vi "SeqMgr.Update Progress.vi"(8 "error in":errorcluster, 9 "Result Info":T1={"State"=enum."PASS", "Code"=0, "Description"=""}, 11 "SeqMgr in":refnum<class "SeqMgr.lvclass">) -> (0 "error out":errorcluster, 1 "Result Info Out":T1={"State"=enum."PASS", "Code"=0, "Description"=""}, 2 "Test State":enum32{"Idle", "Running", "Completed"}(ring), 3 "SeqMgr out":refnum<class "SeqMgr.lvclass">, 4 "New Step":string[](array[string]), 5 "Canceled":bool, 6 "StepCnt":i32)   [LabVIEW 2024, in "EQMF.lvlib" / "SeqMgr.lvlib" / "SeqMgr.lvclass"]
uses:
  SeqMgr.lvclass
  SeqMgr.Result Info.ctl
  SeqMgr.Result State Enum.ctl
  SeqMgr.lvclass/SeqMgr.ctl
  SeqMgr.Progress Type.ctl
  <vilib>/Utility/error.llb/Trim Whitespace One-Sided.vi
  SeqMgr.lvlib
  Strings/String Utils.lvlib
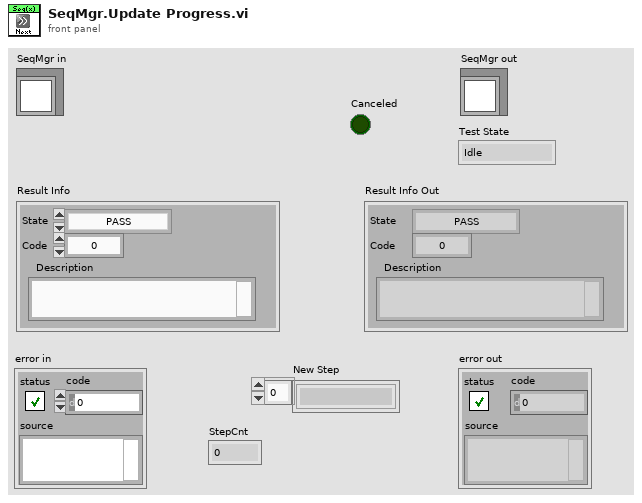
[diagram p1: front panel]
types:
  T1 = typedef "EQMF.lvlib/SeqMgr.lvlib/SeqMgr.Result Info.ctl" = cluster{"State":T2, "Code":i32, "Description":string}
  T2 = typedef "EQMF.lvlib/SeqMgr.lvlib/SeqMgr.Result State Enum.ctl" = enum16{"None", "Passing", "Failing", "PASS", "FAIL", "ABORT", "ERROR"}
  T3 = typedef "EQMF.lvlib/SeqMgr.lvlib/SeqMgr.Progress Type.ctl" = enum16{"Steps", "Time"}
  T4 = typedef "EQMF.lvlib/SeqMgr.lvlib/SeqMgr.Progress Info.ctl" = cluster{"Running":bool, "StartTime":timestamp, "EndTime":timestamp, "Progress":dbl, "Duration(s)":dbl, "ProgType":T3, "StepCnt":i32, "StepTotal":i32, "RemainingTime(s)":dbl, "Test State":enum32{"Idle", "Running", "Completed"}}
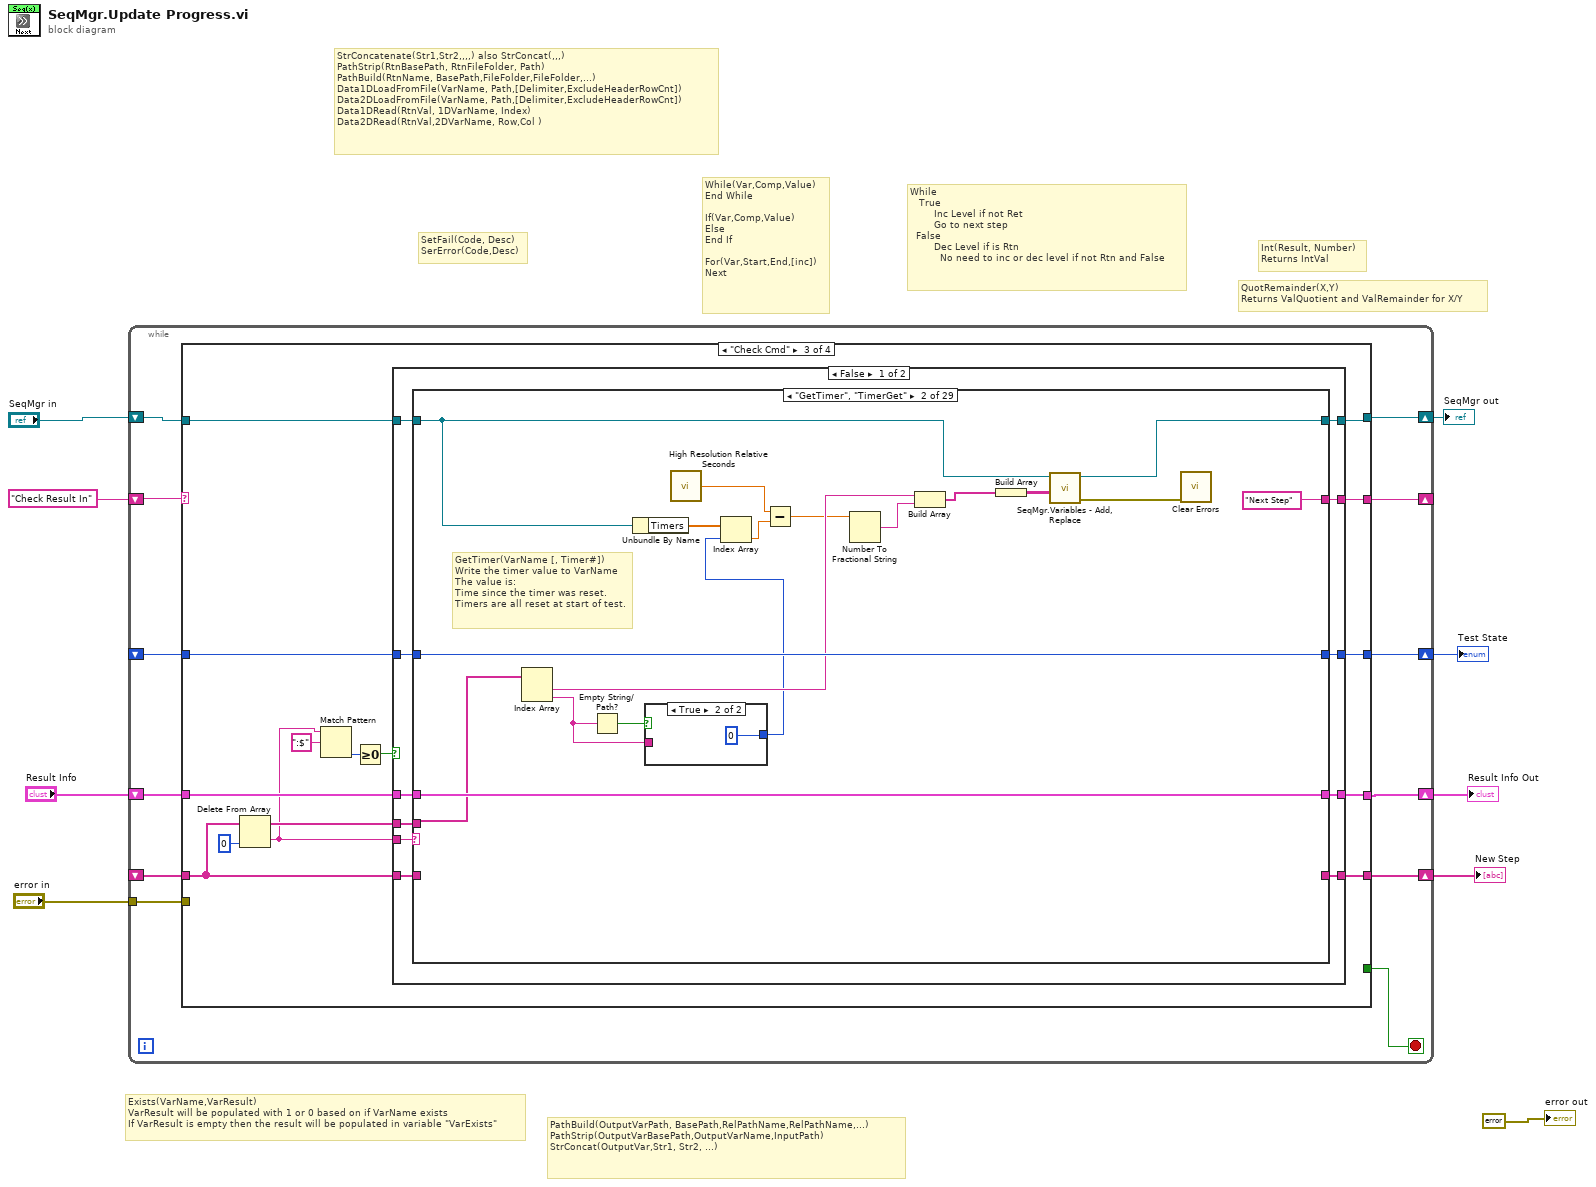
[diagram p0: block diagram]
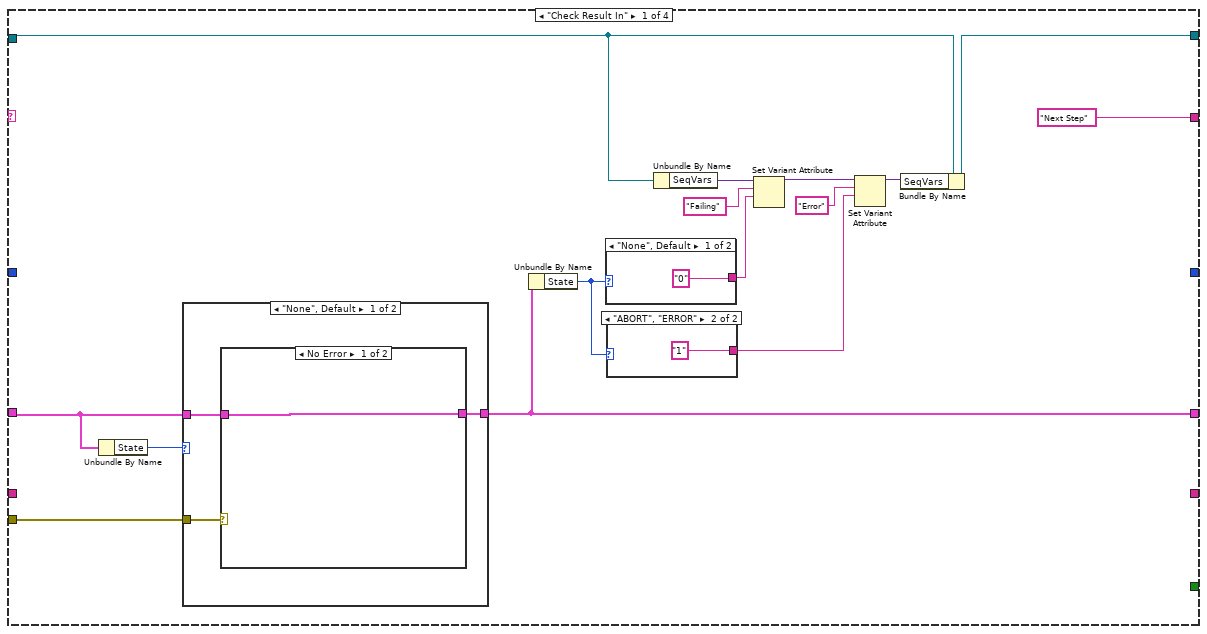
[diagram p2: hidden frame]
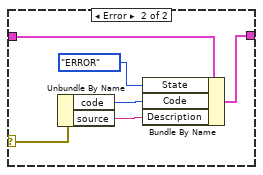
[diagram p3: hidden frame]
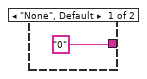
[diagram p5: hidden frame]
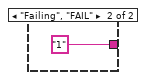
[diagram p6: hidden frame]
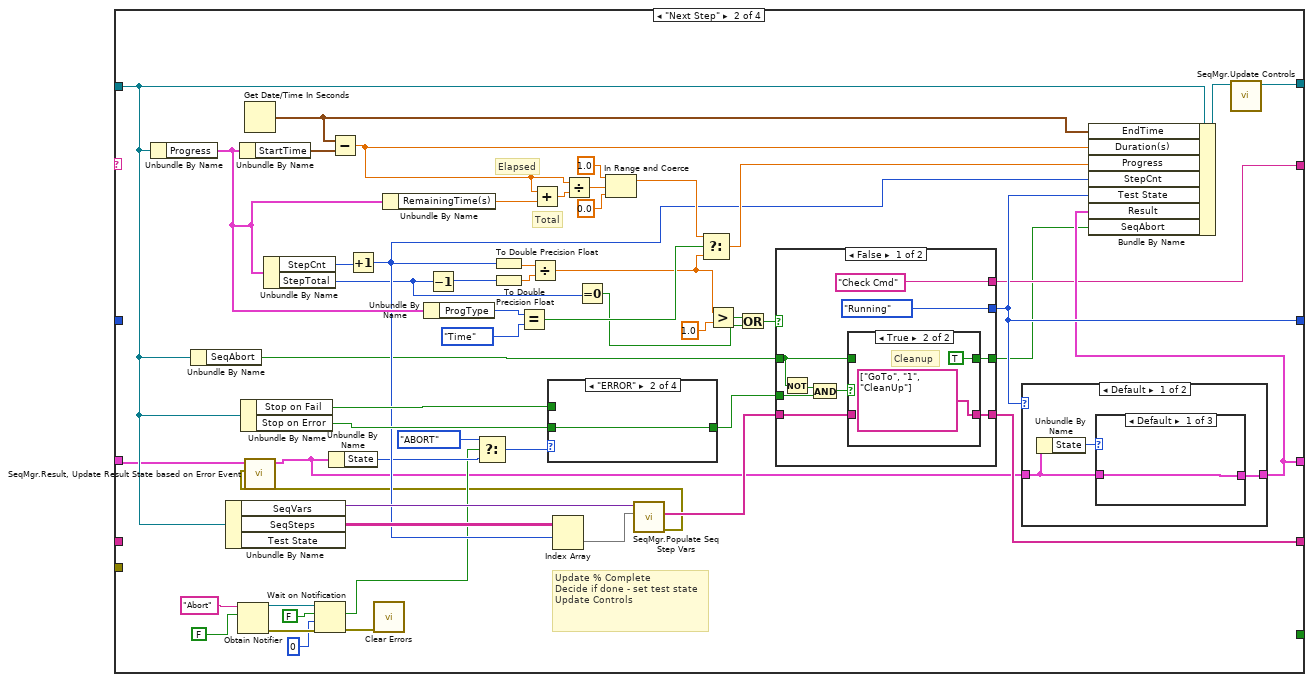
[diagram p7: hidden frame]
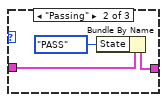
[diagram p8: hidden frame]
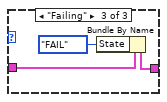
[diagram p9: hidden frame]
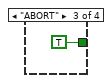
[diagram p12: hidden frame]
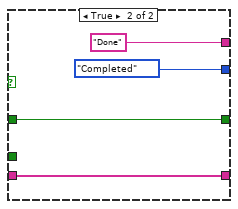
[diagram p15: hidden frame]
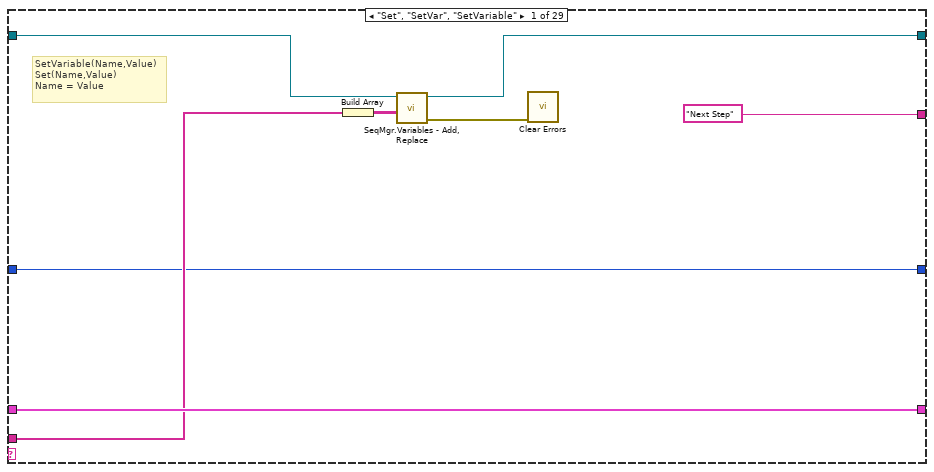
[diagram p16: hidden frame]
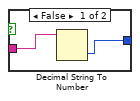
[diagram p17: hidden frame]
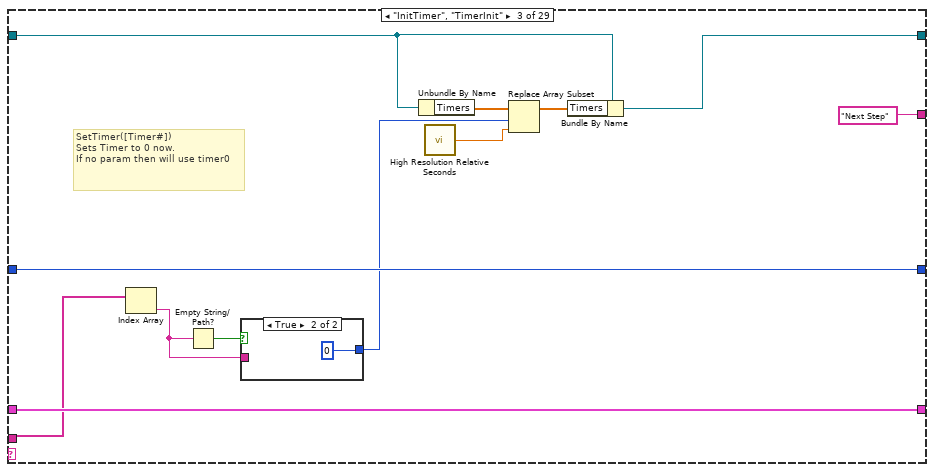
[diagram p18: hidden frame]
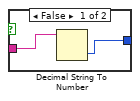
[diagram p19: hidden frame]
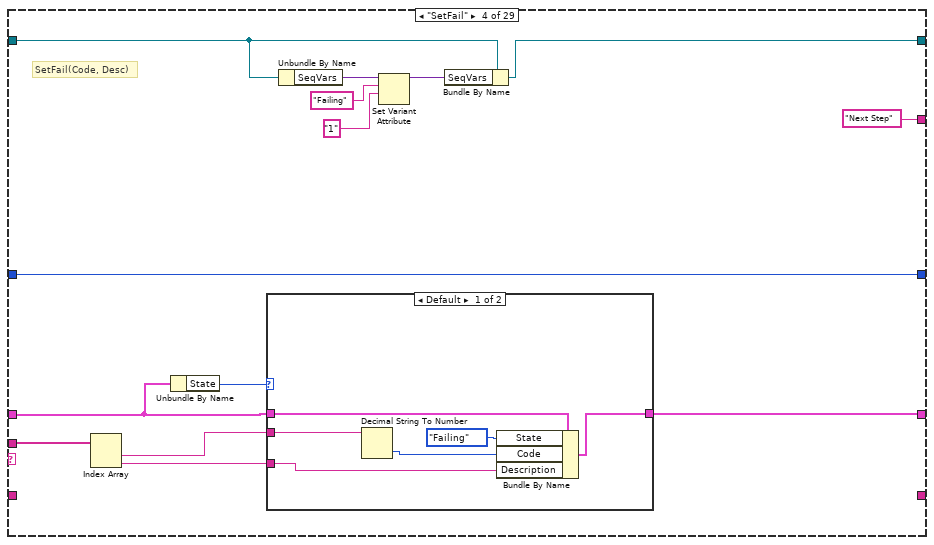
[diagram p20: hidden frame]
diagram:
  # "Exists(VarName,VarResult)\nVarResult will be populated with 1 or 0 based on if VarName exists\nIf VarResult is empty then the result will be populated in variable \"VarExists\""
  # "QuotRemainder(X,Y)\nReturns ValQuotient and ValRemainder for X/Y"
  # "Int(Result, Number)\nReturns IntVal"
  # "StrConcatenate(Str1,Str2,,,,) also StrConcat(,,,)\nPathStrip(RtnBasePath, RtnFileFolder, Path)\nPathBuild(RtnName, BasePath,FileFolder,FileFolder,...)\nData1DLoadFromFile(VarName, Path,[Delimiter,ExcludeHeaderRowCnt])\nData2DLoadFromFile(VarName, Path,[Delimiter,ExcludeHeaderRowCnt])\nData1DRead(RtnVal, 1DVarName, Index)\nData2DRead(RtnVal,2DVarName, Row,Col )"
  # "PathBuild(OutputVarPath, BasePath,RelPathName,RelPathName,...)\nPathStrip(OutputVarBasePath,OutputVarName,InputPath)\nStrConcat(OutputVar,Str1, Str2, ...)"
  # "SetFail(Code, Desc)\nSerError(Code,Desc)"
  # "While\n   True\n        Inc Level if not Ret\n        Go to next step\n  False\n        Dec Level if is Rtn\n          No need to inc or dec level if not Rtn and False"
  # "While(Var,Comp,Value)\nEnd While\n\nIf(Var,Comp,Value)\nElse\nEnd If\n\nFor(Var,Start,End,[inc])\nNext"
  n1 = while {
    shift-right: [w20] -> w8
    shift-left: "SeqMgr in" -> [w21]
    shift-right: [w17] -> w5
    shift-left: "Result Info" -> [w16]
    shift-right: [w13] -> _
    shift-left: "Check Result In" -> [w15]
    tunnel: "error in" -> [w14]
    shift-right: [w19] -> w7
    shift-left: _ -> [w11]
    shift-right: [w18] -> w6
    shift-left: _ -> [w12]
    stop <- w10 stop-if-true
    n2 = case shown="\"Check Cmd\"" w15 {
      tunnel: w21 -> [w32 w67 w152 w914]
      tunnel: [w31 w106 w151 w915] -> w20
      tunnel: [_ w70 w143 w929] -> w19
      tunnel: [_ w105 w146 w930] -> w18
      tunnel: [w27 w104 w145 w916] -> w17
      tunnel: w16 -> [w23 w53 w148 w916]
      tunnel: w14 -> [w36 _ _ _]
      tunnel: ["Next Step" w73 w142 "Done"] -> w13
      tunnel: w12 -> [_ _ w147 w930]
      tunnel: w11 -> [_ _ w144 w929]
      tunnel: [_ _ _ TRUE] -> w10
      frame "Check Result In" {
        n3 = Unbundle By Name(w23) -> ("State"=w22:T2)
        n4 = case shown="\"None\", Default" w22 {
          tunnel: w36 -> [w39 _]
          tunnel: w23 -> [w38 w47]
          tunnel: [w37 w47] -> w27
          frame "None", Default {
            n5 = case shown="No Error" w39 {
              selector: w39 -> [_ w43]
              tunnel: w38 -> [w40 w46]
              tunnel: [w40 w45] -> w37
              frame No Error {
              }
              frame Error {
                n6 = Unbundle By Name(w43) -> ("code"=w42:i32, "source"=w41:string)
                n7 = Bundle By Name(cluster=w46, "State"=SeqMgr.Result_State_Enum."ERROR", "Code"=w42, "Description"=w41) -> (w45:T1)
              }
            }
          }
          frame "ABORT", "ERROR" {
          }
        }
        n8 = Unbundle By Name(w27) -> ("State"=w26:T2)
        n9 = case shown="\"None\", Default" w26 {
          tunnel: ["0" "1"] -> w30
          frame "None", Default {
          }
          frame "Failing", "FAIL" {
          }
        }
        n10 = case shown="\"ABORT\", \"ERROR\"" w26 {
          tunnel: ["0" "1"] -> w25
          frame "None", Default {
          }
          frame "ABORT", "ERROR" {
          }
        }
        n11 = Unbundle By Name(w32) -> ("SeqVars"=w33:variant)
        n12 = Set Variant Attribute(Variant=w33, name="Failing", value=w30) -> (Variant out=w29:variant)  [unwired: 1 in, 2 out]
        n13 = Set Variant Attribute(Variant=w29, name="Error", value=w25) -> (Variant out=w28:variant)  [unwired: 1 in, 2 out]
        n14 = Bundle By Name(cluster=w32, "SeqVars"=w28) -> (w31:refnum<class "SeqMgr.lvclass">)
      }
      frame "Next Step" {
        # "Elapsed"
        # "Total"
        # "Update % Complete\nDecide if done - set test state\nUpdate Controls"
        n15 = Unbundle By Name(w67) -> ("Progress"=w88:T4)
        n16 = Unbundle By Name(w67) -> ("SeqAbort"=w66:bool)
        n17 = Unbundle By Name(w67) -> ("SeqVars"=w79:variant, "SeqSteps"=w87:string[][])  [unwired: 1 out]
        n18 = Obtain Notifier(name (unnamed)="Abort", notification data type=FALSE ("create if not found? (T)")) -> (notifier out=w62:refnum<notifier>, error out=w61:errorcluster)  [unwired: 2 in, 1 out]
        n19 = Unbundle By Name(w88) -> ("StartTime"=w103:timestamp)
        n20 = Unbundle By Name(w67) -> ("Stop on Fail"=w81:bool, "Stop on Error"=w80:bool)
        n21 = Get Date/Time In Seconds() -> (seconds since 1Jan1904=w72:timestamp)
        n22 = Unbundle By Name(w88) -> ("StepCnt"=w89:i32, "StepTotal"=w75:i32)
        n23 = Wait on Notification(notifier=w62, ignore previous (F)=FALSE, timeout in ms (-1)=0, error in (no error)=w61) -> (notification=w55:bool, error out=w60:errorcluster)  [unwired: 2 out]
        n24 = Subtract(x=w72, y=w103) -> (x-y=w102:dbl)
        n25 = Increment(x=w89) -> (x+1=w77:i32)
        n26 = call <vilib>:"Clear Errors.vi"("error in (no error)"=w60) -> ()  [unwired: 5 in, 2 out]
        n27 = Unbundle By Name(w88) -> ("RemainingTime(s)"=w99:dbl)
        n28 = Unbundle By Name(w88) -> ("ProgType"=w93:T3)
        n29 = Decrement(x=w75) -> (x-1=w76:i32)
        n30 = To Double Precision Float(number=w77) -> (double precision float=w100:dbl)
        n31 = To Double Precision Float(number=w76) -> (double precision float=w101:dbl)
        n32 = Equal?(x=w93, y=SeqMgr.Progress_Type."Time" ("ProgType")) -> (x = y?=w91:bool)
        n33 = Divide(x=w100, y=w101) -> (x/y=w86:dbl)
        n34 = Add(x=w102, y=w99) -> (x+y=w98:dbl)
        n35 = Index Array(array=w87, index (row)=w77) -> (element=w78:string[])  [unwired: 1 in]
        n36 = Divide(x=w102, y=w98) -> (x/y=w97:dbl)
        n37 = Equal To 0?(x=w75) -> (x = 0?=w74:bool)
        n38 = In Range and Coerce(upper limit=1.0, x=w97, lower limit=0.0 ("upper limit")) -> (coerced(x)=w94:dbl)  [unwired: 1 out]
        n39 = call "SeqMgr.Populate Seq Step Vars.vi"("Seq Step In"=w78, "Variable Values"=w79) -> ("error out"=w52:errorcluster, "Seq Step Out"=w71:string[])  [unwired: 8 in]
        n40 = call "SeqMgr.Result, Update Result State based on Error Event.vi"("error in"=w52, "Result Info"=w53) -> ("Result Info Out"=w54:T1)  [unwired: 9 in]
        n41 = Unbundle By Name(w54) -> ("State"=w65:T2)
        n42 = Select(t=SeqMgr.Result_State_Enum."ABORT", s=w55, f=w65) -> (s? t:f=w64:T2)
        n43 = case shown="\"ERROR\"" w64 {
          tunnel: w81 -> [w118 _ _ _]
          tunnel: w80 -> [_ w119 _ _]
          tunnel: [w118 w119 TRUE _] -> w69
          frame "Failing", "FAIL" {
          }
          frame "ERROR" {
          }
          frame "ABORT" {
          }
          frame "Passing", Default {
          }
        }
        n44 = Select(t=w94, s=w91, f=w86) -> (s? t:f=w90:dbl)
        n45 = Greater?(x=w86, y=1.0 ("upper limit")) -> (0:w83:bool)
        n46 = Or(x=w83, y=w74) -> (x .or. y?=w84:bool)
        n47 = case shown="False" w84 {
          tunnel: [enum32{"Idle", "Running", "Completed"}."Running" ("Progress.Test State") enum32{"Idle", "Running", "Completed"}."Completed" ("Progress.Test State")] -> w105
          tunnel: ["Check Cmd" "Done"] -> w73
          tunnel: w71 -> [w126 w135]
          tunnel: [w127 w135] -> w70
          tunnel: w69 -> [w125 _]
          tunnel: [w123 w134] -> w68
          tunnel: w66 -> [w121 w134]
          frame False {
            n48 = Not(x=w121) -> (.not. x?=w122:bool)
            n49 = And(x=w122, y=w125) -> (x .and. y?=w124:bool)
            n50 = case shown="True" w124 {
              tunnel: [w131 string[] ["GoTo", "1", "CleanUp"]] -> w127
              tunnel: w126 -> [w131 _]
              tunnel: [w130 TRUE] -> w123
              tunnel: w121 -> [w130 _]
              frame False {
              }
              frame True {
                # "Cleanup"
              }
            }
          }
          frame True {
          }
        }
        n51 = case shown="Default" w105 {
          tunnel: w54 -> [w107 w117]
          tunnel: [w108 w117] -> w104
          frame Default {
            n52 = Unbundle By Name(w107) -> ("State"=w109:T2)
            n53 = case shown="Default" w109 {
              tunnel: [w110 w113 w116] -> w108
              tunnel: w107 -> [w110 w112 w115]
              frame Default {
              }
              frame "Passing" {
                n54 = Bundle By Name(cluster=w112, "State"=SeqMgr.Result_State_Enum."PASS") -> (w113:T1)
              }
              frame "Failing" {
                n55 = Bundle By Name(cluster=w115, "State"=SeqMgr.Result_State_Enum."FAIL") -> (w116:T1)
              }
            }
          }
          frame "Running" {
          }
        }
        n56 = Bundle By Name(cluster=w67, "EndTime"=w72, "Duration(s)"=w102, "Progress"=w90, "StepCnt"=w77, "Test State"=w105, "Result"=w104, "SeqAbort"=w68) -> (w82:refnum<class "SeqMgr.lvclass">)
        n57 = call "SeqMgr.Update Controls.vi"("SeqMgr in"=w82) -> ("SeqMgr out"=w106:refnum<class "SeqMgr.lvclass">)  [unwired: 9 in, 1 out]
      }
      frame "Check Cmd" {
        n58 = Delete From Array(array=w144, index=0) -> (deleted portion=w140:string, array with subset deleted=w149:string[])  [unwired: 1 in]
        n59 = Match Pattern(string=w140, regular expression=":$") -> (offset past match=w139:i32)  [unwired: 1 in, 3 out]
        n60 = Greater Or Equal To 0?(x=w139) -> (x >= 0?=w138:bool)
        n61 = case shown="False" w138 {
          tunnel: w152 -> [w163 w913]
          tunnel: [w162 w913] -> w151
          tunnel: w149 -> [w161 _]
          tunnel: w148 -> [w160 w911]
          tunnel: w147 -> [w159 w912]
          tunnel: [w158 w912] -> w146
          tunnel: [w157 w911] -> w145
          tunnel: w144 -> [w156 w910]
          tunnel: [w155 w910] -> w143
          tunnel: [w154 "Next Step"] -> w142
          tunnel: w140 -> [w153 _]
          frame False {
            n62 = case shown="\"GetTimer\", \"TimerGet\"" w153 {
              tunnel: w163 -> [w168 w181 w196 w215 w236 w255 w270 w284 w305 w312 w319 w356 w385 w422 w479 w495 w529 w599 w614 w707 w722 w755 w768 w783 w811 w833 w861 w897 w908]
              tunnel: [w167 w186 w195 w214 w235 w254 w269 w283 w304 w313 w318 w355 w384 w429 w478 w504 w539 w598 w624 w706 w721 w754 w767 w782 w810 w832 w860 w898 w908] -> w162
              tunnel: w161 -> [w166 w180 w201 w210 w231 w251 w266 w280 w301 w311 w327 w364 w383 w424 _ w494 w534 _ w611 _ w725 w751 w763 w781 w809 w844 w870 w894 _]
              tunnel: w160 -> [w170 w188 w203 w213 w234 w256 w271 w285 w306 w314 w321 w358 w387 w431 w474 w500 w541 w591 w626 w700 w728 w758 w771 w777 w805 w848 w874 w895 w906]
              tunnel: w159 -> [w164 w184 w202 w220 w241 w252 w267 w281 w302 w309 w322 w359 w388 w432 w472 w498 w542 w592 w627 w699 w726 w756 w769 w784 w812 w849 w875 w893 w907]
              tunnel: [w164 w184 w202 w220 w241 w252 w267 w281 w302 w309 w324 w361 w390 w433 w472 w498 w543 w592 w628 w699 w726 w756 w769 w784 w812 w849 w875 w893 w907] -> w158
              tunnel: [w170 w188 w203 w211 w232 w256 w271 w285 w306 w314 w320 w357 w386 w430 w473 w499 w540 w594 w625 w701 w728 w758 w771 w776 w804 w847 w873 w895 w906] -> w157
              tunnel: w156 -> [_ _ _ _ _ _ _ _ _ _ _ _ _ _ _ _ _ _ _ _ _ _ _ _ _ _ _ _ w905]
              tunnel: [_ _ _ _ _ _ _ _ _ _ _ _ _ _ _ _ _ _ _ _ _ _ _ _ _ _ _ _ w905] -> w155
              tunnel: ["Next Step" "Next Step" "Next Step" "Next Step" "Next Step" "Next Step" "Next Step" "Next Step" "Next Step" "Next Step" w328 w365 w393 "Next Step" "Next Step" "Next Step" "Next Step" "Next Step" "Next Step" "Next Step" "Next Step" "Next Step" "Next Step" "Next Step" "Next Step" "Next Step" "Next Step" "Next Step" "Done"] -> w154
              frame "Set", "SetVar", "SetVariable" {
                # "SetVariable(Name,Value)\nSet(Name,Value)\nName = Value"
                n63 = Build Array(w166) -> (w169:string[][])
                n64 = call "SeqMgr.Variables - Add, Replace.vi"("Name, Value"=w169, "SeqMgr in"=w168) -> ("error out"=w165:errorcluster, "SeqMgr out"=w167:refnum<class "SeqMgr.lvclass">)  [unwired: 8 in]
                n65 = call <vilib>:"Clear Errors.vi"("error in (no error)"=w165) -> ()  [unwired: 5 in, 2 out]
              }
              frame "GetTimer", "TimerGet" {
                # "GetTimer(VarName [, Timer#])\nWrite the timer value to VarName\nThe value is:\nTime since the timer was reset.\nTimers are all reset at start of test."
                n66 = Index Array(array=w180) -> (element #1=w176:string, element #2=w178:string)  [unwired: 2 in]
                n67 = Empty String/Path?(string/path=w178) -> (empty?=w179:bool)
                n68 = Unbundle By Name(w181) -> ("Timers"=w177:dbl[])
                n69 = case shown="True" w179 {
                  tunnel: w178 -> [w191 _]
                  tunnel: [w190 0] -> w172
                  frame False {
                    n70 = Decimal String To Number(string=w191) -> (number=w190:i32)  [unwired: 2 in, 1 out]
                  }
                  frame True {
                  }
                }
                n71 = call <vilib>:"High Resolution Relative Seconds.vi"() -> ("relative seconds"=w175:dbl)
                n72 = Index Array(array=w177, index=w172) -> (element=w174:dbl)
                n73 = Subtract(x=w175, y=w174) -> (x-y=w173:dbl)
                n74 = Number To Fractional String(number=w173) -> (F-format string=w182:string)  [unwired: 3 in]
                n75 = Build Array(w176, w182) -> (w183:string[])
                n76 = Build Array(w183) -> (w187:string[][])
                n77 = call "SeqMgr.Variables - Add, Replace.vi"("Name, Value"=w187, "SeqMgr in"=w181) -> ("error out"=w185:errorcluster, "SeqMgr out"=w186:refnum<class "SeqMgr.lvclass">)  [unwired: 8 in]
                n78 = call <vilib>:"Clear Errors.vi"("error in (no error)"=w185) -> ()  [unwired: 5 in, 2 out]
              }
              frame "InitTimer", "TimerInit" {
                # "SetTimer([Timer#])\nSets Timer to 0 now.\nIf no param then will use timer0"
                n79 = Index Array(array=w201) -> (element=w197:string)  [unwired: 1 in]
                n80 = Empty String/Path?(string/path=w197) -> (empty?=w200:bool)
                n81 = case shown="True" w200 {
                  tunnel: w197 -> [w206 _]
                  tunnel: [w205 0] -> w198
                  frame False {
                    n82 = Decimal String To Number(string=w206) -> (number=w205:i32)  [unwired: 2 in, 1 out]
                  }
                  frame True {
                  }
                }
                n83 = Unbundle By Name(w196) -> ("Timers"=w199:dbl[])
                n84 = call <vilib>:"High Resolution Relative Seconds.vi"() -> ("relative seconds"=w193:dbl)
                n85 = Replace Array Subset(array=w199, new element=w193, index=w198) -> (w194:dbl[])
                n86 = Bundle By Name(cluster=w196, "Timers"=w194) -> (w195:refnum<class "SeqMgr.lvclass">)
              }
              frame "SetFail" {
                # "SetFail(Code, Desc)"
                n87 = Index Array(array=w210) -> (element #1=w209:string, element #2=w208:string)  [unwired: 2 in]
                n88 = Unbundle By Name(w213) -> ("State"=w212:T2)
                n89 = case shown="Default" w212 {
                  tunnel: w213 -> [w227 w228]
                  tunnel: [w226 w228] -> w211
                  tunnel: w209 -> [w224 _]
                  tunnel: w208 -> [w223 _]
                  frame Default {
                    n90 = Decimal String To Number(string=w224) -> (number=w222:i32)  [unwired: 2 in, 1 out]
                    n91 = Bundle By Name(cluster=w227, "State"=SeqMgr.Result_State_Enum."Failing", "Code"=w222, "Description"=w223) -> (w226:T1)
                  }
                  frame "Failing", "FAIL", "ERROR" {
                    # "No Change"
                  }
                }
                n92 = Unbundle By Name(w215) -> ("SeqVars"=w217:variant)
                n93 = Set Variant Attribute(Variant=w217, name="Failing", value="1") -> (Variant out=w218:variant)  [unwired: 1 in, 2 out]
                n94 = Bundle By Name(cluster=w215, "SeqVars"=w218) -> (w214:refnum<class "SeqMgr.lvclass">)
              }
              frame "SetError" {
                # "SetError(Code, Desc)"
                n95 = Index Array(array=w231) -> (element #1=w230:string, element #2=w229:string)  [unwired: 2 in]
                n96 = Unbundle By Name(w234) -> ("State"=w233:T2)
                n97 = case shown="Default" w233 {
                  tunnel: w234 -> [w248 w249]
                  tunnel: [w247 w249] -> w232
                  tunnel: w230 -> [w245 _]
                  tunnel: w229 -> [w244 _]
                  frame Default {
                    n98 = Decimal String To Number(string=w245) -> (number=w243:i32)  [unwired: 2 in, 1 out]
                    n99 = Bundle By Name(cluster=w248, "State"=SeqMgr.Result_State_Enum."ERROR", "Code"=w243, "Description"=w244) -> (w247:T1)
                  }
                  frame "ERROR" {
                    # "No Change"
                  }
                }
                n100 = Unbundle By Name(w236) -> ("SeqVars"=w238:variant)
                n101 = Set Variant Attribute(Variant=w238, name="Error", value="1") -> (Variant out=w239:variant)  [unwired: 1 in, 2 out]
                n102 = Bundle By Name(cluster=w236, "SeqVars"=w239) -> (w235:refnum<class "SeqMgr.lvclass">)
              }
              frame "Math" {
                # "Math(Result,Value1,Oper,Value2)\nName = Value Oper Value"
                n103 = call "SeqMgr.Math Statement Execute.vi"("Arguements"=w251) -> ("Vars Out"=w250:string[][])  [unwired: 10 in]
                n104 = call "SeqMgr.Variables - Add, Replace.vi"("Name, Value"=w250, "SeqMgr in"=w255) -> ("error out"=w253:errorcluster, "SeqMgr out"=w254:refnum<class "SeqMgr.lvclass">)  [unwired: 8 in]
                n105 = call <vilib>:"Clear Errors.vi"("error in (no error)"=w253) -> ()  [unwired: 5 in, 2 out]
              }
              frame "Int" {
                n106 = Index Array(array=w266) -> (element #1=w263:string, element #2=w265:string)  [unwired: 2 in]
                n107 = Fract/Exp String To Number(string=w265) -> (number=w259:dbl)  [unwired: 3 in, 1 out]
                n108 = Round To Nearest(number=w259) -> (nearest integer value=w258:dbl)
                n109 = To Long Integer(number=w258) -> (32bit integer=w264:i32)
                n110 = Number To Decimal String(number=w264) -> (decimal integer string=w262:string)  [unwired: 1 in]
                n111 = Build Array(w263, w262) -> (w261:string[])
                n112 = Build Array(w261) -> (w260:string[][])
                n113 = call "SeqMgr.Variables - Add, Replace.vi"("Name, Value"=w260, "SeqMgr in"=w270) -> ("error out"=w268:errorcluster, "SeqMgr out"=w269:refnum<class "SeqMgr.lvclass">)  [unwired: 8 in]
                n114 = call <vilib>:"Clear Errors.vi"("error in (no error)"=w268) -> ()  [unwired: 5 in, 2 out]
              }
              frame "AbsVal" {
                n115 = Index Array(array=w280) -> (element #1=w278:string, element #2=w279:string)  [unwired: 2 in]
                n116 = Fract/Exp String To Number(string=w279) -> (number=w275:dbl)  [unwired: 3 in, 1 out]
                n117 = Absolute Value(x=w275) -> (abs(x)=w274:dbl)
                n118 = call "String.Float to String, No Trailing Zeros.vi"("Numeric"=w274) -> ("String"=w273:string)  [unwired: 10 in]
                n119 = Build Array(w278, w273) -> (w277:string[])
                n120 = Build Array(w277) -> (w276:string[][])
                n121 = call "SeqMgr.Variables - Add, Replace.vi"("Name, Value"=w276, "SeqMgr in"=w284) -> ("error out"=w282:errorcluster, "SeqMgr out"=w283:refnum<class "SeqMgr.lvclass">)  [unwired: 8 in]
                n122 = call <vilib>:"Clear Errors.vi"("error in (no error)"=w282) -> ()  [unwired: 5 in, 2 out]
              }
              frame "QuotRemainder" {
                n123 = Index Array(array=w301) -> (element #1=w300:string, element #2=w297:string)  [unwired: 2 in]
                n124 = Fract/Exp String To Number(string=w297) -> (number=w295:dbl)  [unwired: 3 in, 1 out]
                n125 = Fract/Exp String To Number(string=w300) -> (number=w296:dbl)  [unwired: 3 in, 1 out]
                n126 = Quotient & Remainder(x=w296, y=w295) -> (x-y*floor(x/y)=w294:dbl, floor(x/y)=w292:dbl)
                n127 = To Long Integer(number=w292) -> (32bit integer=w293:i32)
                n128 = Number To Fractional String(number=w294) -> (F-format string=w290:string)  [unwired: 3 in]
                n129 = Number To Decimal String(number=w293) -> (decimal integer string=w291:string)  [unwired: 1 in]
                n130 = Build Array("ValRemainder", w290) -> (w299:string[])
                n131 = Build Array("ValQuotient", w291) -> (w287:string[])
                n132 = Build Array(w299, w287) -> (w298:string[][])
                n133 = call "SeqMgr.Variables - Add, Replace.vi"("Name, Value"=w298, "SeqMgr in"=w305) -> ("error out"=w303:errorcluster, "SeqMgr out"=w304:refnum<class "SeqMgr.lvclass">)  [unwired: 8 in]
                n134 = call <vilib>:"Clear Errors.vi"("error in (no error)"=w303) -> ()  [unwired: 5 in, 2 out]
              }
              frame "SetStopOnFail" {
                # "SetStopOnFail(1 or 0)"
                n135 = Index Array(array=w311) -> (element=w308:string)  [unwired: 1 in]
                n136 = case shown="\"1\", Default" w308 {
                  tunnel: [FALSE TRUE] -> w310
                  frame "0" {
                  }
                  frame "1", Default {
                  }
                }
                n137 = Bundle By Name(cluster=w312, "Stop on Fail"=w310) -> (w313:refnum<class "SeqMgr.lvclass">)
              }
              frame "End", "Exit" {
                # "End(1 or 0)"
                n138 = Index Array(array=w327) -> (element=w326:string)  [unwired: 1 in]
                n139 = Equal?(x=w326, y="1") -> (x = y?=w323:bool)
                n140 = case shown="True" w323 {
                  tunnel: ["Next Step" "Done"] -> w328
                  tunnel: [w331 w338] -> w324
                  tunnel: w322 -> [w331 _]
                  tunnel: w321 -> [w330 w343]
                  tunnel: [w330 w337] -> w320
                  tunnel: w319 -> [w329 w333]
                  tunnel: [w329 w340] -> w318
                  frame False {
                  }
                  frame True {
                    w338 = enum32{"Idle", "Running", "Completed"}."Completed" ("Progress.Test State")
                    n141 = Unbundle By Name(w343) -> ("State"=w342:T2)
                    n142 = Unbundle By Name(w333) -> ("StartTime"=w336:timestamp)
                    n143 = case shown="\"None\", Default" w342 {
                      tunnel: w343 -> [w346 w350 w353 w354]
                      tunnel: [w345 w348 w351 w354] -> w337
                      frame "None", Default {
                        n144 = Bundle By Name(cluster=w346, "State"=SeqMgr.Result_State_Enum."PASS") -> (w345:T1)
                      }
                      frame "Passing" {
                        n145 = Bundle By Name(cluster=w350, "State"=SeqMgr.Result_State_Enum."PASS") -> (w348:T1)
                      }
                      frame "Failing" {
                        n146 = Bundle By Name(cluster=w353, "State"=SeqMgr.Result_State_Enum."FAIL") -> (w351:T1)
                      }
                      frame "PASS".."ABORT" {
                      }
                    }
                    n147 = Get Date/Time In Seconds() -> (seconds since 1Jan1904=w334:timestamp)
                    n148 = Subtract(x=w334, y=w336) -> (x-y=w335:dbl)
                    n149 = Bundle By Name(cluster=w333, "EndTime"=w334, "Duration(s)"=w335, "Progress"=1.0 ("Progress.Progress"), "Test State"=w338, "Result"=w337) -> (w341:refnum<class "SeqMgr.lvclass">)
                    n150 = call "SeqMgr.Update Controls.vi"("SeqMgr in"=w341) -> ("SeqMgr out"=w340:refnum<class "SeqMgr.lvclass">)  [unwired: 9 in, 1 out]
                  }
                }
              }
              frame "CancelTest" {
                # "Cancel(1 or 0)"
                n151 = Index Array(array=w364) -> (element=w363:string)  [unwired: 1 in]
                n152 = Equal?(x=w363, y="1") -> (x = y?=w360:bool)
                n153 = case shown="True" w360 {
                  tunnel: ["Next Step" "Done"] -> w365
                  tunnel: [w368 w377] -> w361
                  tunnel: w359 -> [w368 _]
                  tunnel: w358 -> [w367 w381]
                  tunnel: [w367 w376] -> w357
                  tunnel: w356 -> [w366 w372]
                  tunnel: [w366 w379] -> w355
                  frame False {
                  }
                  frame True {
                    w377 = enum32{"Idle", "Running", "Completed"}."Completed" ("Progress.Test State")
                    n154 = Unbundle By Name(w372) -> ("StartTime"=w375:timestamp)
                    n155 = Get Date/Time In Seconds() -> (seconds since 1Jan1904=w373:timestamp)
                    n156 = Subtract(x=w373, y=w375) -> (x-y=w374:dbl)
                    n157 = Bundle By Name(cluster=w381, "State"=SeqMgr.Result_State_Enum."None") -> (w376:T1)
                    n158 = Bundle By Name(cluster=w372, "TestCanceled"=TRUE, "EndTime"=w373, "Duration(s)"=w374, "Progress"=1.0 ("Progress.Progress"), "Test State"=w377, "Result"=w376) -> (w380:refnum<class "SeqMgr.lvclass">)
                    n159 = call "SeqMgr.Update Controls.vi"("SeqMgr in"=w380) -> ("SeqMgr out"=w379:refnum<class "SeqMgr.lvclass">)  [unwired: 9 in, 1 out]
                  }
                }
              }
              frame "GoTo" {
                # "GoTo(1 or 0,Label)"
                n160 = Index Array(array=w383) -> (element=w392:string)  [unwired: 1 in]
                n161 = Equal?(x=w392, y="0") -> (x = y?=w389:bool)
                n162 = case shown="False" w389 {
                  tunnel: ["Next Step" "Next Step"] -> w393
                  tunnel: [w401 w417] -> w390
                  tunnel: w388 -> [w401 w417]
                  tunnel: w387 -> [w407 w416]
                  tunnel: [w407 w416] -> w386
                  tunnel: w385 -> [w406 w415]
                  tunnel: [w405 w415] -> w384
                  tunnel: w383 -> [w400 _]
                  frame False {
                    n163 = Index Array(array=w400, index=1) -> (element=w398:string)
                    n164 = Unbundle By Name(w406) -> ("StepCnt"=w394:i32, "StepTotal"=w402:i32)
                    n165 = Unbundle By Name(w406) -> ("SeqSteps"=w411:string[][])
                    n166 = Concatenate Strings(w398, ":") -> (w396:string)
                    n167 = To Lower Case(string=w396) -> (all lower case string=w395:string)
                    n168 = Index Array(array=w411, index (col)=0 ("disabled index (col)")) -> (element=w409:string[])  [unwired: 1 in]
                    n169 = To Lower Case(string=w409) -> (all lower case string=w408:string[])
                    n170 = Search 1D Array(1D array=w408, element=w395, start index (0)=w394) -> (index of element=w404:i32)
                    n171 = case shown="-1" w404 {
                      selector: w404 -> [w413 _]
                      tunnel: [w413 w414] -> w403
                      tunnel: w402 -> [_ w414]
                      frame 0, Default {
                      }
                      frame -1 {
                      }
                    }
                    n172 = Bundle By Name(cluster=w406, "StepCnt"=w403) -> (w405:refnum<class "SeqMgr.lvclass">)
                  }
                  frame True {
                  }
                }
              }
              frame "If" {
                n173 = Unbundle By Name(w422) -> ("If Index"=w421:i32[], "StepCnt"=w420:i32)
                n174 = Array Subset(array=w424, index=0, length=3 ("index")) -> (w425:string[])
                n175 = call "SeqMgr.Compare Param Values.vi"("Var,Comp,Var"=w425) -> ("error out"=w419:errorcluster, "Boolean"=w423:bool)  [unwired: 9 in]
                n176 = case shown="False" w423 {
                  tunnel: [w447 w470] -> w433
                  tunnel: w432 -> [w447 w470]
                  tunnel: w431 -> [w440 w471]
                  tunnel: [w439 w471] -> w430
                  tunnel: w422 -> [w438 w468]
                  tunnel: [w442 w467] -> w429
                  tunnel: w424 -> [w444 _]
                  tunnel: w421 -> [w434 w466]
                  tunnel: w420 -> [w436 w465]
                  tunnel: w419 -> [_ _]
                  frame False {
                    # "Sub 1 from Step Cnt\nSince is next step\nWant current step"
                    n177 = Unbundle By Name(w438) -> ("SeqSteps"=w445:string[][], "StepCnt"=w446:i32)
                    n178 = call "SeqMgr.If Statement, Find Else or End.vi"("Arguements"=w444, "Next Step"=w446, "Sequence"=w445) -> ("error out"=w441:errorcluster, "Next Step"=w443:i32, "End"=w435:bool)  [unwired: 6 in]
                    n179 = case shown="False" w435 {
                      tunnel: w438 -> [w451 w455]
                      tunnel: [w450 w455] -> w437
                      tunnel: w436 -> [w449 _]
                      tunnel: w434 -> [w448 _]
                      frame False {
                        n180 = Decrement(x=w449) -> (x-1=w454:i32)
                        n181 = Build Array (concatenate)(w448, w454) -> (w452:i32[])
                        n182 = Array Size(array=w452) -> (size(s)=w453:i32)
                        n183 = Bundle By Name(cluster=w451, "If Index"=w452, "If Level"=w453) -> (w450:refnum<class "SeqMgr.lvclass">)
                      }
                      frame True {
                      }
                    }
                    n184 = case shown="No Error" w441 {
                      selector: w441 -> [_ w459]
                      tunnel: w440 -> [w456 w462]
                      tunnel: [w456 w461] -> w439
                      frame No Error {
                      }
                      frame Error {
                        n185 = Unbundle By Name(w459) -> ("code"=w458:i32, "source"=w457:string)
                        n186 = Bundle By Name(cluster=w462, "State"=SeqMgr.Result_State_Enum."ERROR", "Code"=w458, "Description"=w457) -> (w461:T1)
                      }
                    }
                    n187 = Bundle By Name(cluster=w437, "StepCnt"=w443) -> (w442:refnum<class "SeqMgr.lvclass">)
                  }
                  frame True {
                    # "Inc If Level"
                    n188 = Decrement(x=w465) -> (x-1=w469:i32)
                    n189 = Build Array (concatenate)(w466, w469) -> (w463:i32[])
                    n190 = Array Size(array=w463) -> (size(s)=w464:i32)
                    n191 = Bundle By Name(cluster=w468, "If Index"=w463, "If Level"=w464) -> (w467:refnum<class "SeqMgr.lvclass">)
                  }
                }
              }
              frame "End If" {
                n192 = Unbundle By Name(w479) -> ("If Level"=w485:i32, "If Index"=w482:i32[])
                n193 = Array Size(array=w482) -> (size(s)=w481:i32)
                n194 = Decrement(x=w481) -> (x-1=w476:i32)
                n195 = Less Than 0?(x=w476) -> (x < 0?=w475:bool)
                n196 = Delete From Array(array=w482, length=1, index=w476) -> (array with subset deleted=w480:i32[])  [unwired: 1 out]
                n197 = Decrement(x=w485) -> (x-1=w484:i32)
                n198 = case shown="True" w475 {
                  tunnel: w474 -> [w486 w491]
                  tunnel: [w486 w490] -> w473
                  frame False {
                  }
                  frame True {
                    n199 = Bundle By Name(cluster=w491, "State"=SeqMgr.Result_State_Enum."ERROR", "Code"=-6000, "Description"="Script error.  'End If' is missing an 'If' statement.") -> (w490:T1)
                  }
                }
                n200 = Bundle By Name(cluster=w479, "If Level"=w484, "If Index"=w480) -> (w478:refnum<class "SeqMgr.lvclass">)
              }
              frame "Else" {
                n201 = Unbundle By Name(w495) -> ("SeqSteps"=w497:string[][], "StepCnt"=w496:i32)
                n202 = Unbundle By Name(w495) -> ("If Level"=w510:i32, "If Index"=w507:i32[])
                n203 = Array Size(array=w507) -> (size(s)=w506:i32)
                n204 = call "SeqMgr.If Statement, Find End after Else.vi"("Arguements"=w494, "Next Step"=w496, "Sequence"=w497) -> ("error out"=w493:errorcluster, "Next Step"=w492:i32)  [unwired: 6 in, 1 out]
                n205 = Decrement(x=w506) -> (x-1=w502:i32)
                n206 = Less Than 0?(x=w502) -> (x < 0?=w501:bool)
                n207 = Delete From Array(array=w507, length=1, index=w502) -> (array with subset deleted=w505:i32[])  [unwired: 1 out]
                n208 = Decrement(x=w510) -> (x-1=w509:i32)
                n209 = case shown="No Error" w493 {
                  selector: w493 -> [_ w521]
                  tunnel: w501 -> [w513 _]
                  tunnel: w500 -> [w512 w522]
                  tunnel: [w511 w520] -> w499
                  frame No Error {
                    n210 = case shown="False" w513 {
                      tunnel: w512 -> [w514 w519]
                      tunnel: [w514 w518] -> w511
                      frame False {
                      }
                      frame True {
                        n211 = Bundle By Name(cluster=w519, "State"=SeqMgr.Result_State_Enum."ERROR", "Code"=-6000, "Description"="Script error.  'Else' is missing an 'If' statement.") -> (w518:T1)
                      }
                    }
                  }
                  frame Error {
                    n212 = Unbundle By Name(w521) -> ("code"=w524:i32, "source"=w525:string)
                    n213 = Bundle By Name(cluster=w522, "State"=SeqMgr.Result_State_Enum."ERROR", "Code"=w524, "Description"=w525) -> (w520:T1)
                  }
                }
                n214 = Bundle By Name(cluster=w495, "If Level"=w509, "If Index"=w505, "StepCnt"=w492) -> (w504:refnum<class "SeqMgr.lvclass">)
              }
              frame "While" {
                n215 = Unbundle By Name(w529) -> ("WRet"=w530:bool, "While Index"=w532:i32[], "StepCnt"=w531:i32, "While Level"=w526:i32)
                n216 = Bundle By Name(cluster=w529, "WRet"=FALSE ("FlowCtrl.WRet")) -> (w528:refnum<class "SeqMgr.lvclass">)
                n217 = Array Subset(array=w534, index=0, length=3 ("index")) -> (w535:string[])
                n218 = call "SeqMgr.Compare Param Values.vi"("Var,Comp,Var"=w535) -> ("Boolean"=w533:bool)  [unwired: 9 in, 1 out]
                n219 = case shown="False" w533 {
                  tunnel: [w557 w580] -> w543
                  tunnel: w542 -> [w557 w580]
                  tunnel: w541 -> [w547 w581]
                  tunnel: [w546 w581] -> w540
                  tunnel: w528 -> [w551 w578]
                  tunnel: [w552 w577] -> w539
                  tunnel: w534 -> [w554 _]
                  tunnel: w532 -> [w550 w576]
                  tunnel: w531 -> [_ w575]
                  tunnel: w530 -> [w545 w579]
                  tunnel: w526 -> [w544 _]
                  frame False {
                    n220 = Unbundle By Name(w551) -> ("SeqSteps"=w555:string[][], "StepCnt"=w556:i32)
                    n221 = case shown="True" w545 {
                      tunnel: w551 -> [w565 w568]
                      tunnel: w550 -> [_ w566]
                      tunnel: [w565 w569] -> w549
                      tunnel: w544 -> [_ w567]
                      frame False {
                      }
                      frame True {
                        # "Dec Level"
                        n222 = Array Size(array=w566) -> (size(s)=w572:i32)
                        n223 = Decrement(x=w572) -> (x-1=w570:i32)
                        n224 = Delete From Array(array=w566, length=1, index=w570) -> (array with subset deleted=w571:i32[])  [unwired: 1 out]
                        n225 = Decrement(x=w567) -> (x-1=w574:i32)
                        n226 = Bundle By Name(cluster=w568, "While Level"=w574, "While Index"=w571) -> (w569:refnum<class "SeqMgr.lvclass">)
                      }
                    }
                    n227 = call "SeqMgr.While Statement, Find End.vi"("Arguements"=w554, "Next Step"=w556, "Sequence"=w555) -> ("error out"=w548:errorcluster, "Next Step"=w553:i32)  [unwired: 6 in, 1 out]
                    n228 = case shown="No Error" w548 {
                      selector: w548 -> [_ w561]
                      tunnel: w547 -> [w558 w564]
                      tunnel: [w558 w563] -> w546
                      frame No Error {
                      }
                      frame Error {
                        n229 = Unbundle By Name(w561) -> ("code"=w560:i32, "source"=w559:string)
                        n230 = Bundle By Name(cluster=w564, "State"=SeqMgr.Result_State_Enum."ERROR", "Code"=w560, "Description"=w559) -> (w563:T1)
                      }
                    }
                    n231 = Bundle By Name(cluster=w549, "StepCnt"=w553) -> (w552:refnum<class "SeqMgr.lvclass">)
                  }
                  frame True {
                    # "Sub 1 from Step Cnt\nSince is next step\nWant current step"
                    n232 = case shown="False" w579 {
                      tunnel: w578 -> [w586 w589]
                      tunnel: [w585 w589] -> w577
                      tunnel: w576 -> [w583 _]
                      tunnel: w575 -> [w582 _]
                      frame False {
                        # "Increment Level"
                        n233 = Decrement(x=w582) -> (x-1=w584:i32)
                        n234 = Build Array (concatenate)(w583, w584) -> (w587:i32[])
                        n235 = Array Size(array=w587) -> (size(s)=w588:i32)
                        n236 = Bundle By Name(cluster=w586, "While Index"=w587, "While Level"=w588) -> (w585:refnum<class "SeqMgr.lvclass">)
                      }
                      frame True {
                        # "Is returned from End While.  Stay at current level"
                      }
                    }
                  }
                }
              }
              frame "End While" {
                # "Go back to 'While' statement"
                n237 = Unbundle By Name(w599) -> ("While Index"=w601:i32[])
                n238 = Array Size(array=w601) -> (size(s)=w600:i32)
                n239 = Decrement(x=w600) -> (x-1=w593:i32)
                n240 = Less Than 0?(x=w593) -> (x < 0?=w595:bool)
                n241 = Index Array(array=w601, index=w593) -> (element=w596:i32)
                n242 = case shown="True" w595 {
                  tunnel: w591 -> [w602 w607]
                  tunnel: [w602 w606] -> w594
                  frame False {
                  }
                  frame True {
                    n243 = Bundle By Name(cluster=w607, "State"=SeqMgr.Result_State_Enum."ERROR", "Code"=-6000, "Description"="Script error.  'End While' is missing a 'While' statement.") -> (w606:T1)
                  }
                }
                n244 = Bundle By Name(cluster=w599, "WRet"=TRUE ("FlowCtrl.WRet"), "StepCnt"=w596) -> (w598:refnum<class "SeqMgr.lvclass">)
              }
              frame "For" {
                n245 = Unbundle By Name(w614) -> ("FRet"=w615:bool, "For Index"=w621:i32[], "StepCnt"=w620:i32, "For Level"=w617:i32)
                n246 = call "SeqMgr.Variables - Get.vi"("SeqMgr in"=w614) -> ("Vars"=w613:variant)  [unwired: 8 in, 2 out]
                n247 = Index Array(array=w611, index=5) -> (element=w610:string)
                n248 = Bundle By Name(cluster=w614, "FRet"=FALSE ("FlowCtrl.WRet")) -> (w619:refnum<class "SeqMgr.lvclass">)
                n249 = Get Variant Attribute(Variant=w613, name=w610, default value (empty Variant)="") -> (value=w608:string)  [unwired: 1 in, 3 out]
                n250 = case shown="True" w615 {
                  tunnel: w611 -> [w630 w636]
                  tunnel: [TRUE ("Continue") w635] -> w622
                  tunnel: [w629 w634] -> w616
                  tunnel: w608 -> [_ w633]
                  frame False {
                    n251 = Index Array(array=w630, index=1) -> (element=w629:string)
                  }
                  frame True {
                    n252 = Replace Array Subset(array=w636, new element=w633, index=0) -> (w637:string[])
                    n253 = call "SeqMgr.For Loop Compare Values.vi"("Var,Start,End,Inc"=w637) -> ("Counter New Val"=w634:string, "Continue"=w635:bool)  [unwired: 8 in, 1 out]
                  }
                }
                n254 = case shown="False" w622 {
                  tunnel: [w658 w688] -> w628
                  tunnel: w627 -> [w658 w688]
                  tunnel: w626 -> [w650 w689]
                  tunnel: [w649 w689] -> w625
                  tunnel: w619 -> [w654 w686]
                  tunnel: [w645 w680] -> w624
                  tunnel: w611 -> [w640 w678]
                  tunnel: w621 -> [w653 w685]
                  tunnel: w620 -> [_ w684]
                  tunnel: w615 -> [w648 w687]
                  tunnel: w617 -> [w647 _]
                  tunnel: w616 -> [w641 w676]
                  frame False {
                    n255 = Unbundle By Name(w654) -> ("SeqSteps"=w656:string[][], "StepCnt"=w657:i32)
                    n256 = case shown="False" w648 {
                      tunnel: w654 -> [w666 w669]
                      tunnel: w653 -> [_ w667]
                      tunnel: [w666 w670] -> w652
                      tunnel: w647 -> [_ w668]
                      frame False {
                      }
                      frame True {
                        # "Dec Level"
                        n257 = Array Size(array=w667) -> (size(s)=w673:i32)
                        n258 = Decrement(x=w673) -> (x-1=w671:i32)
                        n259 = Delete From Array(array=w667, length=1, index=w671) -> (array with subset deleted=w672:i32[])  [unwired: 1 out]
                        n260 = Decrement(x=w668) -> (x-1=w675:i32)
                        n261 = Bundle By Name(cluster=w669, "For Level"=w675, "For Index"=w672) -> (w670:refnum<class "SeqMgr.lvclass">)
                      }
                    }
                    n262 = Index Array(array=w640, index=5) -> (element=w643:string)
                    n263 = Build Array(w643, w641) -> (w644:string[])
                    n264 = Build Array(w644) -> (w639:string[][])
                    n265 = call "SeqMgr.For Statement, Find Next.vi"("Arguements"=w640, "Next Step"=w657, "Sequence"=w656) -> ("error out"=w651:errorcluster, "Next Step"=w655:i32)  [unwired: 6 in, 1 out]
                    n266 = case shown="Error" w651 {
                      selector: w651 -> [_ w662]
                      tunnel: w650 -> [w659 w665]
                      tunnel: [w659 w664] -> w649
                      frame No Error {
                      }
                      frame Error {
                        n267 = Unbundle By Name(w662) -> ("code"=w661:i32, "source"=w660:string)
                        n268 = Bundle By Name(cluster=w665, "State"=SeqMgr.Result_State_Enum."ERROR", "Code"=w661, "Description"=w660) -> (w664:T1)
                      }
                    }
                    n269 = Bundle By Name(cluster=w652, "StepCnt"=w655) -> (w646:refnum<class "SeqMgr.lvclass">)
                    n270 = call "SeqMgr.Variables - Add, Replace.vi"("Name, Value"=w639, "SeqMgr in"=w646) -> ("SeqMgr out"=w645:refnum<class "SeqMgr.lvclass">)  [unwired: 8 in, 1 out]
                  }
                  frame True {
                    # "For,Var,Start,End,Inc"
                    # "Sub 1 from Step Cnt\nSince is next step\nWant current step"
                    n271 = case shown="False" w687 {
                      tunnel: w686 -> [w694 w697]
                      tunnel: [w693 w697] -> w679
                      tunnel: w685 -> [w691 _]
                      tunnel: w684 -> [w690 _]
                      frame False {
                        # "Increment Level"
                        n272 = Decrement(x=w690) -> (x-1=w692:i32)
                        n273 = Build Array (concatenate)(w691, w692) -> (w695:i32[])
                        n274 = Array Size(array=w695) -> (size(s)=w696:i32)
                        n275 = Bundle By Name(cluster=w694, "For Index"=w695, "For Level"=w696) -> (w693:refnum<class "SeqMgr.lvclass">)
                      }
                      frame True {
                        # "Is returned from Next.  Stay at current level"
                      }
                    }
                    n276 = Index Array(array=w678, index=5) -> (element=w683:string)
                    n277 = Build Array(w683, w676) -> (w682:string[])
                    n278 = Build Array(w682) -> (w681:string[][])
                    n279 = call "SeqMgr.Variables - Add, Replace.vi"("Name, Value"=w681, "SeqMgr in"=w679) -> ("SeqMgr out"=w680:refnum<class "SeqMgr.lvclass">)  [unwired: 8 in, 1 out]
                  }
                }
              }
              frame "Next" {
                # "Go back to 'For' statement"
                n280 = Unbundle By Name(w707) -> ("For Index"=w709:i32[])
                n281 = Array Size(array=w709) -> (size(s)=w708:i32)
                n282 = Decrement(x=w708) -> (x-1=w702:i32)
                n283 = Less Than 0?(x=w702) -> (x < 0?=w703:bool)
                n284 = Index Array(array=w709, index=w702) -> (element=w704:i32)
                n285 = case shown="True" w703 {
                  tunnel: w700 -> [w710 w715]
                  tunnel: [w710 w714] -> w701
                  frame False {
                  }
                  frame True {
                    n286 = Bundle By Name(cluster=w715, "State"=SeqMgr.Result_State_Enum."ERROR", "Code"=-6000, "Description"="Script error.  'Next' is missing a 'For' statement.") -> (w714:T1)
                  }
                }
                n287 = Bundle By Name(cluster=w707, "StepCnt"=w704, "FRet"=TRUE ("FlowCtrl.FRet")) -> (w706:refnum<class "SeqMgr.lvclass">)
              }
              frame "PathBuild" {
                n288 = Delete From Array(array=w725, index=0) -> (deleted portion=w716:string, array with subset deleted=w723:string[])  [unwired: 1 in]
                n289 = for {
                  shift-right: [w732] -> w720
                  shift-left: _ -> [w731]
                  tunnel: w723 -> [w730] mode=indexing
                  i -> [w733]
                  n290 = call <vilib>:"Trim Whitespace.vi"("string"=w730) -> ("trimmed string"=w729:string)  [unwired: 1 in]
                  n291 = case shown="1, Default" w733 {
                    tunnel: w729 -> [w734 w742]
                    tunnel: [w735 w741] -> w732
                    tunnel: w731 -> [w736 _]
                    frame 1, Default {
                      n292 = case shown="\"\"" w734 {
                        selector: w734 -> [_ w738]
                        tunnel: w736 -> [w737 w740]
                        tunnel: [w737 w739] -> w735
                        frame "" {
                          # "Skip empty"
                        }
                        frame Default {
                          n293 = Build Path(base path=w740, name or relative path=w738) -> (appended path=w739:path)
                        }
                      }
                    }
                    frame 0 {
                      n294 = String To Path(string=w742) -> (path=w741:path)
                    }
                  }
                }
                n295 = Path To String(path=w720) -> (string=w719:string)
                n296 = Build Array(w716, w719) -> (w718:string[])
                n297 = Build Array(w718) -> (w717:string[][])
                n298 = call "SeqMgr.Variables - Add, Replace.vi"("Name, Value"=w717, "SeqMgr in"=w722) -> ("SeqMgr out"=w721:refnum<class "SeqMgr.lvclass">)  [unwired: 8 in, 1 out]
              }
              frame "PathStrip" {
                # "PathStrip(VarNameBasePath, VarNameTopName, Path)"
                n299 = Index Array(array=w751) -> (element #1=w750:string, element #2=w749:string, element #3=w744:string)  [unwired: 3 in]
                n300 = String To Path(string=w744) -> (path=w743:path)
                n301 = Strip Path(path=w743) -> (stripped path=w748:path, name=w747:string)
                n302 = Path To String(path=w748) -> (string=w746:string)
                n303 = Build Array(w750, w746) -> (w753:string[])
                n304 = Build Array(w749, w747) -> (w745:string[])
                n305 = Build Array(w753, w745) -> (w752:string[][])
                n306 = call "SeqMgr.Variables - Add, Replace.vi"("Name, Value"=w752, "SeqMgr in"=w755) -> ("SeqMgr out"=w754:refnum<class "SeqMgr.lvclass">)  [unwired: 8 in, 1 out]
              }
              frame "StrConcat", "StrConcatenate" {
                n307 = Delete From Array(array=w763, index=0) -> (deleted portion=w762:string, array with subset deleted=w759:string[])  [unwired: 1 in]
                n308 = for {
                  shift-right: [w774] -> w760
                  shift-left: "" -> [w773]
                  tunnel: w759 -> [w772] mode=indexing
                  n309 = Concatenate Strings(w773, w772) -> (w774:string)
                }
                n310 = Build Array(w762, w760) -> (w766:string[])
                n311 = Build Array(w766) -> (w765:string[][])
                n312 = call "SeqMgr.Variables - Add, Replace.vi"("Name, Value"=w765, "SeqMgr in"=w768) -> ("SeqMgr out"=w767:refnum<class "SeqMgr.lvclass">)  [unwired: 8 in, 1 out]
              }
              frame "Data2DLoadFromFile" {
                # "Line Feed\nCarriage Return\nLF\nor\nCR\nor\nCRLF"
                # "Data2DLoadFromFile(VarName,RtnMaxRow,RtnMaxCol,Path,[ColDelim,HeaderCnt])"
                n313 = call "SeqMgr.Data 2D Load from File.vi"("Args"=w781) -> ("error out"=w778:errorcluster, "Max Indices"=w775:string[][], "Data"=w779:string[][], "Name"=w780:string)  [unwired: 7 in]
                n314 = case shown="No Error" w778 {
                  tunnel: w783 -> [w801 w802]
                  tunnel: [w795 w802] -> w782
                  tunnel: w780 -> [w798 _]
                  tunnel: w779 -> [w794 _]
                  tunnel: w775 -> [w793 _]
                  frame No Error {
                    n315 = To Variant(anything=w794) -> (Variant=w797:variant)
                    n316 = Unbundle By Name(w801) -> ("Data2D"=w800:variant)
                    n317 = Set Variant Attribute(Variant=w800, name=w798, value=w797) -> (Variant out=w799:variant)  [unwired: 1 in, 2 out]
                    n318 = Bundle By Name(cluster=w801, "Data2D"=w799) -> (w796:refnum<class "SeqMgr.lvclass">)
                    n319 = call "SeqMgr.Variables - Add, Replace.vi"("Name, Value"=w793, "SeqMgr in"=w796) -> ("SeqMgr out"=w795:refnum<class "SeqMgr.lvclass">)  [unwired: 8 in, 1 out]
                  }
                  frame Error {
                  }
                }
                n320 = case shown="No Error" w778 {
                  selector: w778 -> [_ w791]
                  tunnel: w777 -> [w786 w787]
                  tunnel: [w786 w788] -> w776
                  frame No Error {
                  }
                  frame Error {
                    n321 = Unbundle By Name(w791) -> ("code"=w790:i32, "source"=w789:string)
                    n322 = Bundle By Name(cluster=w787, "State"=SeqMgr.Result_State_Enum."ERROR", "Code"=w790, "Description"=w789) -> (w788:T1)
                  }
                }
              }
              frame "Data1DLoadFromFile" {
                # "Line Feed\nCarriage Return\nLF\nor\nCR\nor\nCRLF"
                # "Data1DLoadFromFile(VarName,RtnMaxIndex,Path,[ColDelim,HeaderCnt])"
                n323 = call "SeqMgr.Data 1D Load from File.vi"("Args"=w809) -> ("error out"=w806:errorcluster, "Max Indices"=w803:string[][], "Data"=w807:string[], "Name"=w808:string)  [unwired: 7 in]
                n324 = case shown="No Error" w806 {
                  tunnel: w811 -> [w829 w830]
                  tunnel: [w823 w830] -> w810
                  tunnel: w808 -> [w826 _]
                  tunnel: w807 -> [w824 _]
                  tunnel: w803 -> [w821 _]
                  frame No Error {
                    n325 = To Variant(anything=w824) -> (Variant=w825:variant)
                    n326 = Unbundle By Name(w829) -> ("Data1D"=w828:variant)
                    n327 = Set Variant Attribute(Variant=w828, name=w826, value=w825) -> (Variant out=w827:variant)  [unwired: 1 in, 2 out]
                    n328 = Bundle By Name(cluster=w829, "Data1D"=w827) -> (w822:refnum<class "SeqMgr.lvclass">)
                    n329 = call "SeqMgr.Variables - Add, Replace.vi"("Name, Value"=w821, "SeqMgr in"=w822) -> ("SeqMgr out"=w823:refnum<class "SeqMgr.lvclass">)  [unwired: 8 in, 1 out]
                  }
                  frame Error {
                  }
                }
                n330 = case shown="Error" w806 {
                  selector: w806 -> [_ w819]
                  tunnel: w805 -> [w814 w815]
                  tunnel: [w814 w816] -> w804
                  frame No Error {
                  }
                  frame Error {
                    n331 = Unbundle By Name(w819) -> ("code"=w818:i32, "source"=w817:string)
                    n332 = Bundle By Name(cluster=w815, "State"=SeqMgr.Result_State_Enum."ERROR", "Code"=w818, "Description"=w817) -> (w816:T1)
                  }
                }
              }
              frame "Data2DRead" {
                # "Data2DRead(RtnVal,2DVarName, Row,Col )"
                n333 = Index Array(array=w844) -> (element #1=w837:string, element #2=w834:string, element #3=w842:string, element #4=w841:string)  [unwired: 4 in]
                n334 = Decimal String To Number(string=w842) -> (number=w840:i32)  [unwired: 2 in, 1 out]
                n335 = Decimal String To Number(string=w841) -> (number=w839:i32)  [unwired: 2 in, 1 out]
                n336 = Unbundle By Name(w833) -> ("Data2D"=w846:variant)
                n337 = Get Variant Attribute(Variant=w846, name=w834, default value (empty Variant)=string[][] [] ("Data")) -> (found=w835:bool, value=w843:string[][])  [unwired: 1 in, 2 out]
                n338 = case shown="False" w835 {
                  tunnel: w848 -> [w855 w858]
                  tunnel: [w856 w858] -> w847
                  tunnel: w834 -> [w852 _]
                  frame False {
                    n339 = Format Into String(format string="Array variable \"%s\" not found.", w852) -> (resulting string=w851:string)  [unwired: 2 in, 1 out]
                    n340 = Bundle By Name(cluster=w855, "State"=SeqMgr.Result_State_Enum."ERROR", "Code"=-5000, "Description"=w851) -> (w856:T1)
                  }
                  frame True {
                  }
                }
                n341 = Index Array(array=w843, index (row)=w840, index (col)=w839) -> (element=w838:string)
                n342 = Build Array(w837, w838) -> (w836:string[])
                n343 = Build Array(w836) -> (w831:string[][])
                n344 = call "SeqMgr.Variables - Add, Replace.vi"("Name, Value"=w831, "SeqMgr in"=w833) -> ("SeqMgr out"=w832:refnum<class "SeqMgr.lvclass">)  [unwired: 8 in, 1 out]
              }
              frame "Data1DRead" {
                # "Data1DRead(RtnVal, 1DVarName, Index)"
                n345 = Index Array(array=w870) -> (element #1=w865:string, element #2=w862:string, element #3=w868:string)  [unwired: 3 in]
                n346 = Decimal String To Number(string=w868) -> (number=w867:i32)  [unwired: 2 in, 1 out]
                n347 = Unbundle By Name(w861) -> ("Data1D"=w872:variant)
                n348 = Get Variant Attribute(Variant=w872, name=w862, default value (empty Variant)=string[] [] ("Data")) -> (found=w863:bool, value=w869:string[])  [unwired: 1 in, 2 out]
                n349 = case shown="False" w863 {
                  tunnel: w874 -> [w881 w884]
                  tunnel: [w882 w884] -> w873
                  tunnel: w862 -> [w878 _]
                  frame False {
                    n350 = Format Into String(format string="Array variable \"%s\" not found.", w878) -> (resulting string=w877:string)  [unwired: 2 in, 1 out]
                    n351 = Bundle By Name(cluster=w881, "State"=SeqMgr.Result_State_Enum."ERROR", "Code"=-5000, "Description"=w877) -> (w882:T1)
                  }
                  frame True {
                  }
                }
                n352 = Index Array(array=w869, index=w867) -> (element=w866:string)
                n353 = Build Array(w865, w866) -> (w864:string[])
                n354 = Build Array(w864) -> (w859:string[][])
                n355 = call "SeqMgr.Variables - Add, Replace.vi"("Name, Value"=w859, "SeqMgr in"=w861) -> ("SeqMgr out"=w860:refnum<class "SeqMgr.lvclass">)  [unwired: 8 in, 1 out]
              }
              frame "Exists" {
                # "Exists(VarName,VarResult)\nVarResult will be populated with 1 or 0 based on if VarName exists\nIf VarResult is empty then the result will be populated in variable \"VarExists\""
                n356 = Index Array(array=w894) -> (element #1=w886:string, element #2=w887:string)  [unwired: 2 in]
                n357 = Unbundle By Name(w897) -> ("SeqVars"=w901:variant)
                n358 = case shown="\"\"" w887 {
                  selector: w887 -> [w902 _]
                  tunnel: [w902 "VarExists"] -> w885
                  frame Default {
                  }
                  frame "" {
                  }
                }
                n359 = Get Variant Attribute(Variant=w901, name=w886, default value (empty Variant)="" ("String")) -> (found=w891:bool)  [unwired: 1 in, 3 out]
                n360 = Select(t="1", s=w891, f="0") -> (s? t:f=w888:string)
                n361 = Build Array(w885, w888) -> (w900:string[])
                n362 = Build Array(w900) -> (w899:string[][])
                n363 = call "SeqMgr.Variables - Add, Replace.vi"("Name, Value"=w899, "SeqMgr in"=w897) -> ("SeqMgr out"=w898:refnum<class "SeqMgr.lvclass">)  [unwired: 8 in, 1 out]
              }
              frame Default {
                # "This command is not handled internally.\nReturn to sequence state"
              }
            }
          }
          frame True {
            # "This is a label.\nSkip it and go to next step."
          }
        }
      }
      frame "Done", Default {
        n364 = Unbundle By Name(w916) -> ("State"=w919:T2)
        n365 = case shown="\"Failing\", \"FAIL\"" w919 {
          tunnel: ["0" "1" "1"] -> w922
          frame "None", Default {
          }
          frame "Failing", "FAIL" {
          }
          frame "ERROR" {
          }
        }
        n366 = case shown="\"ABORT\", \"ERROR\"" w919 {
          tunnel: ["0" "1"] -> w918
          frame "None", Default {
          }
          frame "ABORT", "ERROR" {
          }
        }
        n367 = Unbundle By Name(w914) -> ("SeqVars"=w923:variant)
        n368 = Set Variant Attribute(Variant=w923, name="Failing", value=w922) -> (Variant out=w921:variant)  [unwired: 1 in, 2 out]
        n369 = Set Variant Attribute(Variant=w921, name="Error", value=w918) -> (Variant out=w920:variant)  [unwired: 1 in, 2 out]
        n370 = Bundle By Name(cluster=w914, "SeqVars"=w920) -> (w915:refnum<class "SeqMgr.lvclass">)
        n371 = Unbundle By Name(w915) -> ("TestCanceled"=→"Canceled":bool, "StepCnt"=→"StepCnt":i32)
      }
    }
  }
  "SeqMgr out" <- w8
  "New Step" <- w7
  "Test State" <- w6
  "Result Info Out" <- w5
  "error out" <- errorcluster {"status"=FALSE, "code"=0, "source"=""} ("error out")
